vi "Day 15.1.vi"(11 "String":string) -> (3 "sum":u64)   [LabVIEW 2021]
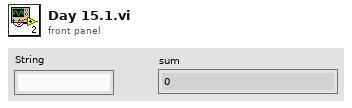
[diagram p1: front panel]
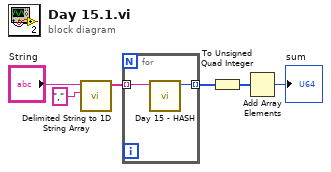
[diagram p0: block diagram]
diagram:
  n1 = call <vilib>:"Delimited String to 1D String Array.vi"("delimiter"=",", "delimited string"="String") -> ("string array"=w4:string[])  [unwired: 9 in]
  n2 = for {
    tunnel: w4 -> [w8] mode=indexing
    tunnel: [w7] -> w2 mode=indexing
    n3 = call "Day 15 - HASH.vi"("String"=w8) -> ("HASH"=w7:i32)  [unwired: 10 in]
  }
  n4 = To Unsigned Quad Integer(1:w2) -> (0:w1:u64[])
  n5 = Add Array Elements(numeric array=w1) -> (sum=→"sum":u64)
